vi "Example - setup and read wavelength.vi"() -> ()   [LabVIEW 2009]
doc: "Sample program that starts the wavelength meter server, sets a few appopriate options, and then reads the current wavelength until the user hits 'stop'."
panel:
  in  "stop":bool
  out "result":dbl
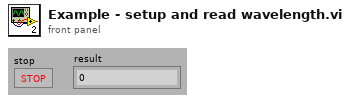
[diagram p1: front panel]
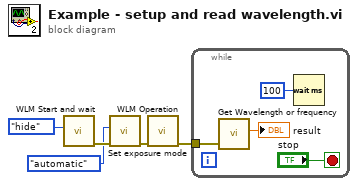
[diagram p0: block diagram]
diagram:
  n1 = call "WLM Start and wait.vi"("command (show)"=enum16{"show", "hide", "exit"}."hide") -> ("error out"=w5:errorcluster)  [unwired: 1 in, 9 out]
  n2 = call "Set exposure mode.vi"("error in (no error)"=w5, "exposure mode"=enum16{"automatic", "manual"}."automatic") -> ("error out"=w4:errorcluster)  [unwired: 9 out]
  n3 = call "WLM Operation.vi"("error in (no error)"=w4) -> ("error out"=w1:errorcluster)  [unwired: 1 in, 9 out]
  n4 = while {
    tunnel: w1 -> [w9]
    stop <- "stop" stop-if-true
    n5 = call "Get Wavelength or frequency.vi"("error in (no error)"=w9) -> ("result"=→"result":dbl)  [unwired: 2 in, 8 out]
    n6 = Wait (ms)(milliseconds to wait=u32 100) -> ()  [unwired: 1 out]
  }
